vi "Clousure.vi"(8 "error in (no error)":errorcluster, 11 "ConcreteCreatorA in":refnum<class "ConcreteCreatorA.lvclass">) -> (0 "error out":errorcluster, 3 "ConcreteCreatorA out":refnum<class "ConcreteCreatorA.lvclass">)   [LabVIEW 2020, in "FactoryMethod.lvlib" / "ConcreteCreatorA.lvclass"]
uses:
  ConcreteCreatorA.lvclass
  Creator/Creator.lvclass
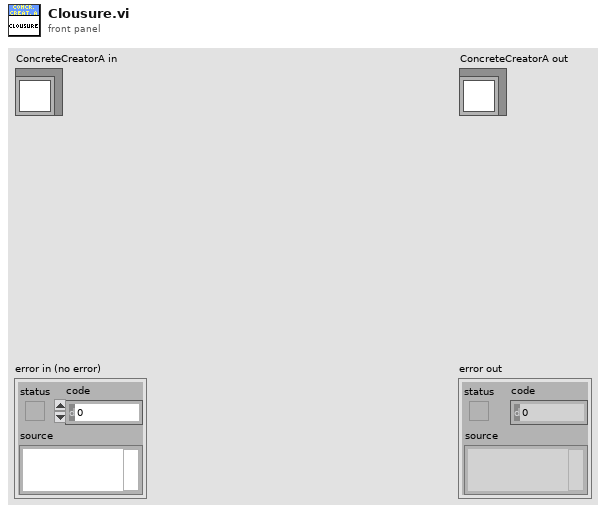
[diagram p1: front panel]
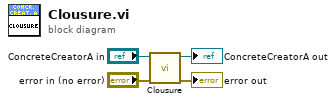
[diagram p0: block diagram]
diagram:
  n1 = call-parent "Clousure.vi"("error in (no error)"="error in (no error)", "Creator in"="ConcreteCreatorA in") -> ("error out"=→"error out":errorcluster, "Creator out"=→"ConcreteCreatorA out":refnum<class "ConcreteCreatorA.lvclass">)  [unwired: 8 in]
